vi "Main.vi"() -> ()   [LabVIEW 2020]
uses:
  Tank Class/Tank.lvclass
  Pump Class/Pump.lvclass
  Sensor Class/Sensor.lvclass
  Sensor Class/Sensor.lvclass/Sensor.ctl
  Pump Class/Pump.lvclass/Pump.ctl
  Tank Class/Tank.lvclass/Tank.ctl
panel:
  out "Level 2":bool
  out "Level 1":bool
  out "Pump":bool
  in  "stop":bool
  out "Tank":dbl(slide) scale=0.0..100.0
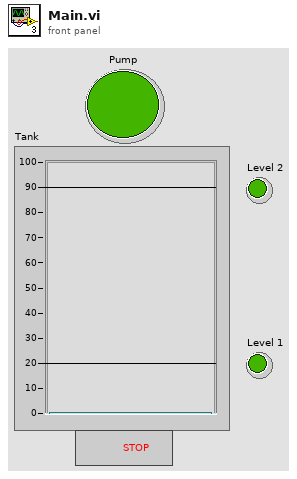
[diagram p1: front panel]
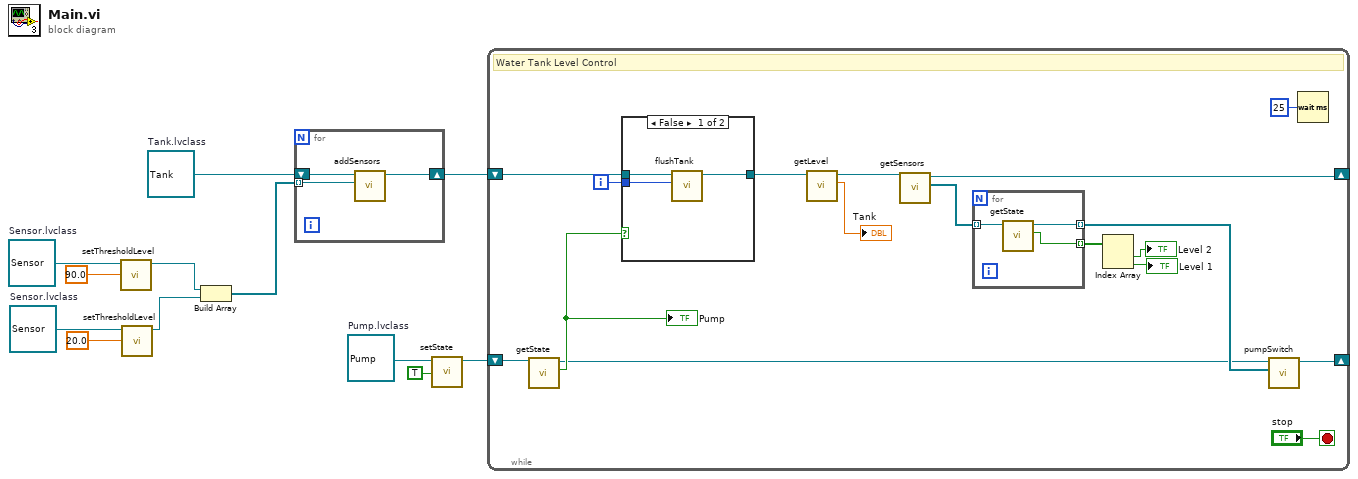
[diagram p0: block diagram]
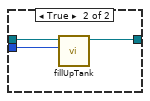
[diagram p2: hidden frame]
diagram:
  w3 = refnum<class "Sensor.lvclass"> refnum  # Sensor.lvclass
  w7 = refnum<class "Pump.lvclass"> refnum  # Pump.lvclass
  w11 = refnum<class "Sensor.lvclass"> refnum  # Sensor.lvclass
  w12 = refnum<class "Tank.lvclass"> refnum  # Tank.lvclass
  n1 = call "setThresholdLevel.vi"("Threshold Level"=90.0, "Sensor in"=w11) -> ("Sensor out"=w1:refnum<class "Sensor.lvclass">)  [unwired: 8 in, 1 out]
  n2 = call "setThresholdLevel.vi"("Threshold Level"=20.0, "Sensor in"=w3) -> ("Sensor out"=w2:refnum<class "Sensor.lvclass">)  [unwired: 8 in, 1 out]
  n3 = Build Array(w1, w2) -> (w8:refnum<class "Sensor.lvclass">[])
  n4 = for {
    shift-right: [w14] -> w10
    shift-left: w12 -> [w15]
    tunnel: w8 -> [w13] mode=indexing
    n5 = call "addSensors.vi"("Sensor.lvclass"=w13, "Tank in"=w15) -> ("Tank out"=w14:refnum<class "Tank.lvclass">)  [unwired: 8 in, 1 out]
  }
  n6 = call "setState.vi"("state"=TRUE, "Pump in"=w7) -> ("Pump out"=w6:refnum<class "Pump.lvclass">)  [unwired: 8 in, 1 out]
  n7 = while {
    shift-right: [w30] -> _
    shift-left: w6 -> [w31]
    shift-right: [w24] -> _
    shift-left: w10 -> [w29]
    i -> [w23]
    stop <- "stop" stop-if-true
    # "Water Tank Level Control"
    n8 = call "getState.vi"("Pump in"=w31) -> ("state"=w20:bool, "Pump out"=w19:refnum<class "Pump.lvclass">)  [unwired: 8 in, 1 out]
    "Pump" <- w20
    n9 = case shown="False" w20 {
      tunnel: [w34 w38] -> w18
      tunnel: w29 -> [w35 w37]
      tunnel: w23 -> [w33 w36]
      frame False {
        n10 = call "flushTank.vi"("Index"=w33, "Tank in"=w35) -> ("Tank out"=w34:refnum<class "Tank.lvclass">)  [unwired: 8 in, 1 out]
      }
      frame True {
        n11 = call "fillUpTank.vi"("Index"=w36, "Tank in"=w37) -> ("Tank out"=w38:refnum<class "Tank.lvclass">)  [unwired: 8 in, 1 out]
      }
    }
    n12 = call "getLevel.vi"("Tank in"=w18) -> ("Level"=→"Tank":dbl, "Tank out"=w22:refnum<class "Tank.lvclass">)  [unwired: 8 in, 1 out]
    n13 = call "getSensors.vi"("Tank in"=w22) -> ("Sensors"=w32:refnum<class "Sensor.lvclass">[], "Tank out"=w24:refnum<class "Tank.lvclass">)  [unwired: 8 in, 1 out]
    n14 = for {
      tunnel: w32 -> [w41] mode=indexing
      tunnel: [w40] -> w27 mode=indexing
      tunnel: [w39] -> w26 mode=indexing
      n15 = call "getState.vi"("Sensor in"=w41) -> ("State"=w39:bool, "Sensor out"=w40:refnum<class "Sensor.lvclass">)  [unwired: 8 in, 1 out]
    }
    n16 = Index Array(array=w26) -> (element #1=→"Level 2":bool, element #2=→"Level 1":bool)  [unwired: 2 in]
    n17 = call "pumpSwitch.vi"("Sensors"=w27, "Pump in"=w19) -> ("Pump out"=w30:refnum<class "Pump.lvclass">)  [unwired: 8 in, 1 out]
    n18 = Wait (ms)(milliseconds to wait=u32 25) -> ()  [unwired: 1 out]
  }
